vi "Move to Motor.vi"(2 "Turn":dbl, 3 "Forward":dbl) -> (0 "Right":dbl, 1 "Left":dbl)   [LabVIEW 2017]
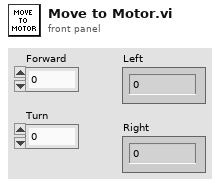
[diagram p1: front panel]
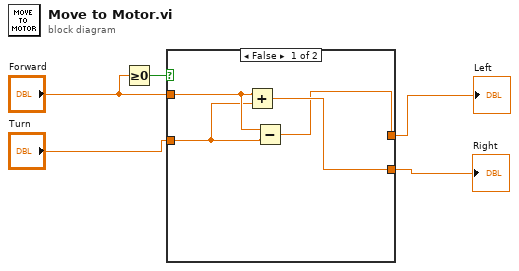
[diagram p0: block diagram]
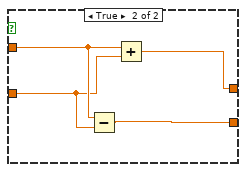
[diagram p2: hidden frame]
diagram:
  n1 = Greater Or Equal To 0?(x="Forward") -> (x >= 0?=w1:bool)
  n2 = case shown="False" w1 {
    tunnel: "Forward" -> [w8 w11]
    tunnel: "Turn" -> [w7 w10]
    tunnel: [w6 w13] -> w4
    tunnel: [w9 w12] -> w5
    frame False {
      n3 = Add(x=w8, y=w7) -> (x+y=w9:dbl)
      n4 = Subtract(x=w8, y=w7) -> (x-y=w6:dbl)
    }
    frame True {
      n5 = Subtract(x=w11, y=w10) -> (x-y=w12:dbl)
      n6 = Add(x=w11, y=w10) -> (x+y=w13:dbl)
    }
  }
  "Left" <- w4
  "Right" <- w5
